vi "DeleteCells.vi"(0 "Column in":refnum<class "Column.lvclass">, 5 "Cell Position":T1, 9 "Table CtlRef In":refnum<vi>, 11 "error in (no error)":errorcluster, 12 "# Rows":i32) -> (4 "Column out":refnum<class "Column.lvclass">, 10 "Table CtlRef Out":refnum<vi>, 15 "error out":errorcluster)   [LabVIEW 2013, in "Column.lvclass"]
doc: "Intended to be used as part of Delete Row(s) function, this method only shifts formatting. Values can be more efficiently deleted by row with array functions.\n\nThe funcitonality was made column-specific so that SingleVal can be handled appropriately."
uses:
  Column.lvclass
  <vilib>/Utility/miscctls.llb/LVRowAndColumnTypeDef.ctl
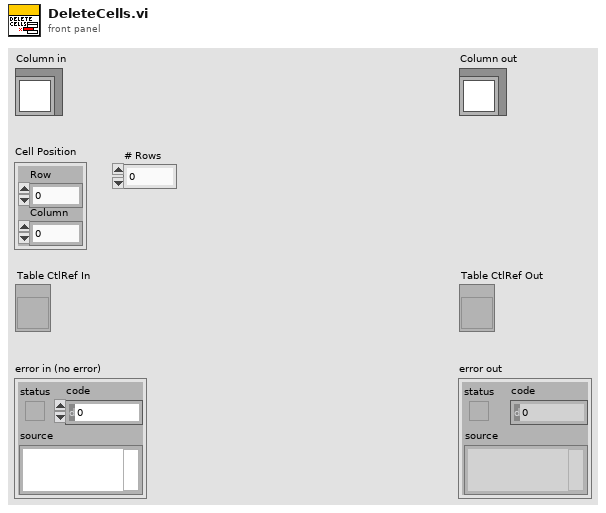
[diagram p1: front panel]
types:
  T1 = typedef "LVRowAndColumnTypeDef.ctl" = cluster{"Row":i32, "Column":i32}
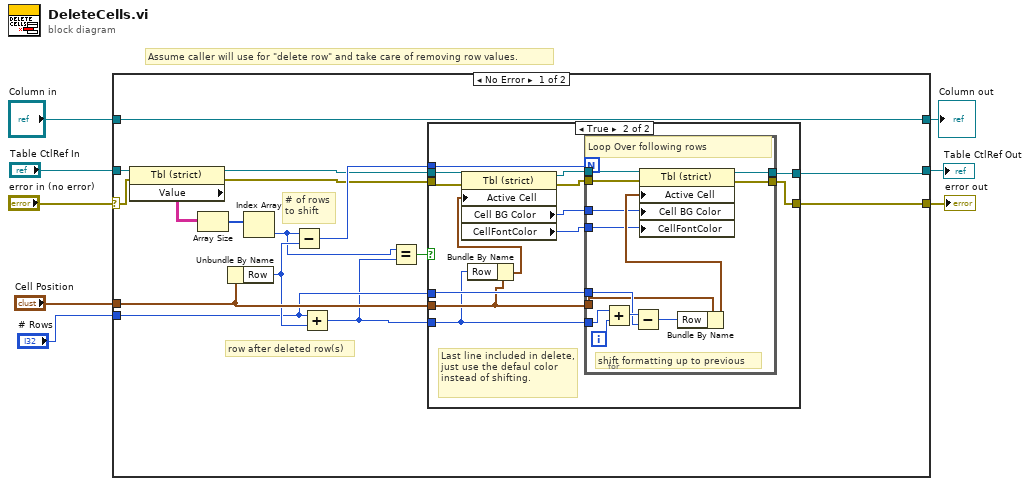
[diagram p0: block diagram]
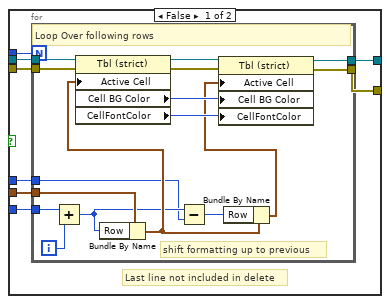
[diagram p2: hidden frame]
diagram:
  # "Assume caller will use for \"delete row\" and take care of removing row values."
  n1 = case shown="No Error" "error in (no error)" {
    selector: "error in (no error)" -> [w15 w77]
    tunnel: [w9 w77] -> w2
    tunnel: [w24 w76] -> w7
    tunnel: "Column in" -> [w24 w76]
    tunnel: "Table CtlRef In" -> [w17 w75]
    tunnel: [w20 w75] -> w3
    tunnel: "Cell Position" -> [w21 _]
    tunnel: "# Rows" -> [w18 _]
    frame No Error {
      # "row after deleted row(s)"
      # "# of rows\nto shift"
      n2 = property class="Tbl (strict)"(reference=w17, error in=w15) -> (reference out=w16:refnum<vi>, error out=w14:errorcluster, "Value"=w13:string[][])
      n3 = Array Size(array=w13) -> (size(s)=w23:i32[])
      n4 = Unbundle By Name(w21) -> ("Row"=w19:i32)
      n5 = Index Array(array=w23) -> (element=w10:i32)  [unwired: 1 in]
      n6 = Subtract(x=w10, y=w19) -> (x-y=w22:i32)
      n7 = Add(x=w18, y=w19) -> (x+y=w11:i32)
      n8 = Equal?(x=w10, y=w11) -> (x = y?=w12:bool)
      n9 = case shown="True" w12 {
        tunnel: w22 -> [w32 w60]
        tunnel: w11 -> [w31 w49]
        tunnel: w21 -> [w30 w53]
        tunnel: [w29 w51] -> w20
        tunnel: [w28 w50] -> w9
        tunnel: w18 -> [w27 w61]
        tunnel: w16 -> [w26 w59]
        tunnel: w14 -> [w25 w56]
        frame False {
          # "Last line not included in delete"
          n10 = for {
            N: w32 -> [_]
            tunnel: w26 -> [w45]
            tunnel: w25 -> [w44]
            tunnel: w31 -> [w48]
            tunnel: w30 -> [w46]
            tunnel: [w41] -> w29
            tunnel: [w40] -> w28
            tunnel: w27 -> [w33]
            i -> [w47]
            # "shift formatting up to previous"
            # "Loop Over following rows"
            n11 = Add(x=w48, y=w47) -> (x+y=w34:i32)
            n12 = Bundle By Name(cluster=w46, "Row"=w34) -> (w35:T1)
            n13 = property class="Tbl (strict)"(reference=w45, error in=w44, "Active Cell"=w35) -> (reference out=w43:refnum<vi>, error out=w42:errorcluster, "Cell BG Color"=w39:u32, "CellFontColor"=w38:u32)
            n14 = Subtract(x=w34, y=w33) -> (x-y=w37:i32)
            n15 = Bundle By Name(cluster=w35, "Row"=w37) -> (w36:T1)
            n16 = property class="Tbl (strict)"(reference=w43, error in=w42, "Active Cell"=w36, "Cell BG Color"=w39, "CellFontColor"=w38) -> (reference out=w41:refnum<vi>, error out=w40:errorcluster)
          }
        }
        frame True {
          # "Last line included in delete, just use the defaul color instead of shifting."
          n17 = Bundle By Name(cluster=w53, "Row"=w49) -> (w52:T1)
          n18 = property class="Tbl (strict)"(reference=w59, error in=w56, "Active Cell"=w52) -> (reference out=w58:refnum<vi>, error out=w57:errorcluster, "Cell BG Color"=w55:u32, "CellFontColor"=w54:u32)
          n19 = for {
            N: w60 -> [_]
            tunnel: w58 -> [w66]
            tunnel: w57 -> [w65]
            tunnel: w53 -> [w67]
            tunnel: [w73] -> w51
            tunnel: [w72] -> w50
            tunnel: w61 -> [w68]
            tunnel: w55 -> [w64]
            tunnel: w54 -> [w63]
            tunnel: w49 -> [w62]
            i -> [w74]
            # "shift formatting up to previous"
            # "Loop Over following rows"
            n20 = Add(x=w62, y=w74) -> (x+y=w69:i32)
            n21 = Subtract(x=w69, y=w68) -> (x-y=w71:i32)
            n22 = Bundle By Name(cluster=w67, "Row"=w71) -> (w70:T1)
            n23 = property class="Tbl (strict)"(reference=w66, error in=w65, "Active Cell"=w70, "Cell BG Color"=w64, "CellFontColor"=w63) -> (reference out=w73:refnum<vi>, error out=w72:errorcluster)
          }
        }
      }
    }
    frame Error {
    }
  }
  "error out" <- w2
  "Column out" <- w7
  "Table CtlRef Out" <- w3
